vi "Random Competition.vi"() -> ()   [LabVIEW 2024]
panel:
  out "Points B":dbl
  out "Points A":dbl
  out "Winner 3":bool
  out "Tie":bool
  out "Winner A":bool
  out "Random Number B":dbl
  out "Random Number A":dbl
  in  "Number of Iterations":i32
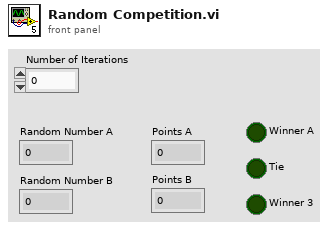
[diagram p1: front panel]
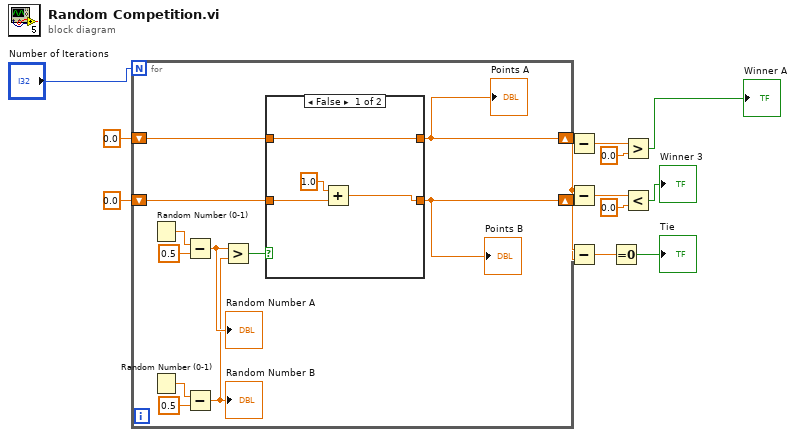
[diagram p0: block diagram]
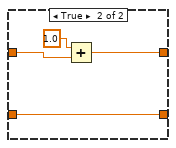
[diagram p2: hidden frame]
diagram:
  n1 = for {
    N: "Number of Iterations" -> [_]
    shift-right: [w14] -> w1
    shift-left: 0.0 -> [w16]
    shift-right: [w15] -> w2
    shift-left: 0.0 -> [w17]
    n2 = Random Number (0-1)() -> (number: 0 to 1=w22:dbl)
    n3 = Random Number (0-1)() -> (number: 0 to 1=w24:dbl)
    n4 = Subtract(x=w22, y=0.5) -> (x-y=w20:dbl)
    "Random Number A" <- w20
    n5 = Subtract(x=w24, y=0.5) -> (x-y=w19:dbl)
    "Random Number B" <- w19
    n6 = Greater?(x=w20, y=w19) -> (0:w18:bool)
    n7 = case shown="False" w18 {
      tunnel: [w25 w31] -> w15
      tunnel: w17 -> [w25 w30]
      tunnel: [w26 w29] -> w14
      tunnel: w16 -> [w27 w29]
      frame False {
        n8 = Add(x=1.0, y=w27) -> (x+y=w26:dbl)
      }
      frame True {
        n9 = Add(x=1.0, y=w30) -> (x+y=w31:dbl)
      }
    }
    "Points A" <- w15
    "Points B" <- w14
  }
  n10 = Subtract(x=w2, y=w1) -> (x-y=w8:dbl)
  n11 = Subtract(x=w2, y=w1) -> (x-y=w5:dbl)
  n12 = Subtract(x=w2, y=w1) -> (x-y=w10:dbl)
  n13 = Equal To 0?(x=w10) -> (x = 0?=→"Tie":bool)
  n14 = Greater?(x=w8, y=0.0) -> (0:→"Winner A":bool)
  n15 = Less?(x=w5, y=0.0) -> (x < y?=→"Winner 3":bool)
